vi "Add.vi"(7 "Service VI? (F)":bool, 8 "error in (no error)":errorcluster, 9 "RESTful VI configuration":T1={"Service VI Type"=enum."Web Method", "Load VI at statup"=TRUE, "Keep VI in memory"=TRUE, "Output type"=enum."Terminal", "Output format"=enum."XML", "Use headers"=TRUE, "Buffered"=TRUE, "eng_Load VI by name"=FALSE}, 10 "ProjectItem Refnum":refnum<vi>, 11 "NI_AB_API_RESTful in":refnum<class "NI_AB_API_RESTful.lvclass">) -> (0 "error out":errorcluster, 3 "NI_AB_API_RESTful out":refnum<class "NI_AB_API_RESTful.lvclass">)   [LabVIEW 2020, in "NI_AB_API_RESTful.lvclass"]
uses:
  <vilib>/AppBuilder/AB_API/RESTful/NI_AB_API_RESTful.lvclass
  <vilib>/AppBuilder/AB_API/RESTful/NI_AB_API_RESTful.lvclass/NI_AB_API_RESTful.ctl
  <vilib>/AppBuilder/AB_Classes/Build/AB_Build.lvclass
  <vilib>/AppBuilder/AB_Classes/Source/AB_Source.lvclass
  <vilib>/AppBuilder/AB_API/Build/NI_AB_API_Build.lvclass
  <vilib>/AppBuilder/AB_Classes/RESTful/AB_RESTfulWebService.lvclass
  e:/builds/penguin/labview/branches/2020/dev/dist/vi.lib/AppBuilder/AB_API/Targetfile/NI_AB_API_Targetfile.lvclass
  e:/builds/penguin/labview/branches/2020/dev/dist/vi.lib/AppBuilder/AB_API/Build/NI_AB_API_Build.lvclass
  e:/builds/penguin/labview/branches/2020/dev/dist/vi.lib/AppBuilder/AB_API/RESTful/NI_AB_API_RESTful.lvclass
  e:/builds/penguin/labview/branches/2020/dev/dist/vi.lib/AppBuilder/AB_Classes/WebService/AB_WebService.lvclass
  e:/builds/penguin/labview/branches/2020/dev/dist/vi.lib/AppBuilder/AB_Classes/TargetFile/AB_Targetfile.lvclass
  e:/builds/penguin/labview/branches/2020/dev/dist/vi.lib/AppBuilder/AB_Classes/Build/AB_Build.lvclass
  e:/builds/penguin/labview/branches/2020/dev/dist/vi.lib/AppBuilder/AB_Classes/RESTful/AB_RESTfulWebService.lvclass
  <vilib>/AppBuilder/AB_Classes/Source/VI/AB_Source_VI.lvclass
  e:/builds/penguin/labview/branches/2020/dev/dist/vi.lib/AppBuilder/AB_Classes/Source/AB_Source.lvclass
  e:/builds/penguin/labview/branches/2020/dev/dist/vi.lib/AppBuilder/AB_Classes/Source/VI/AB_Source_VI.lvclass
  <vilib>/AppBuilder/AB_Classes/Source/RESTfulVI/Configure_RESTfulVI/AB_RESTful_VIType.ctl
  <vilib>/AppBuilder/AB_Classes/Source/RESTfulVI/Configure_RESTfulVI/AB_RESTful_OutputType.ctl
  <vilib>/AppBuilder/AB_Classes/Source/RESTfulVI/Configure_RESTfulVI/AB_RESTful_OutputFormat.ctl
  <vilib>/AppBuilder/AB_Classes/Source/RESTfulVI/Configure_RESTfulVI/AB_RESTful_Configuration.ctl
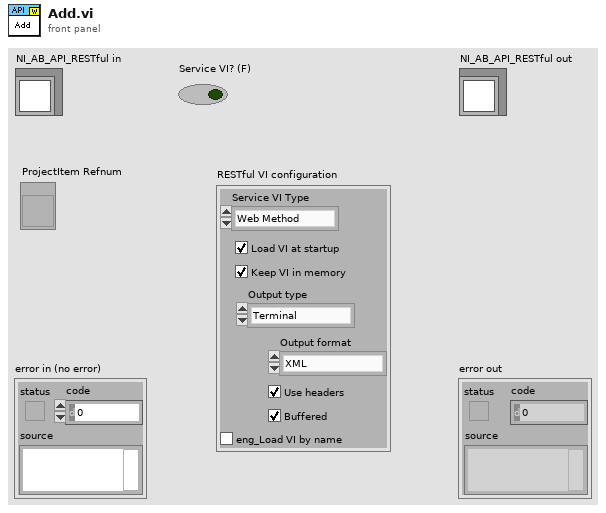
[diagram p1: front panel]
types:
  T1 = typedef "AB_RESTful_Configuration.ctl" = cluster{"Service VI Type":T2, "Load VI at statup":bool, "Keep VI in memory":bool, "Output type":T3, "Output format":T4, "Use headers":bool, "Buffered":bool, "eng_Load VI by name":bool}
  T2 = typedef "AB_RESTful_VIType.ctl" = enum32{"Web Method", "Auxiliary", "eng_Internal", "eng_Content"}
  T3 = typedef "AB_RESTful_OutputType.ctl" = enum32{"Terminal", "Stream"}
  T4 = typedef "AB_RESTful_OutputFormat.ctl" = enum32{"XML", "Text", "HTML", "JSON"}
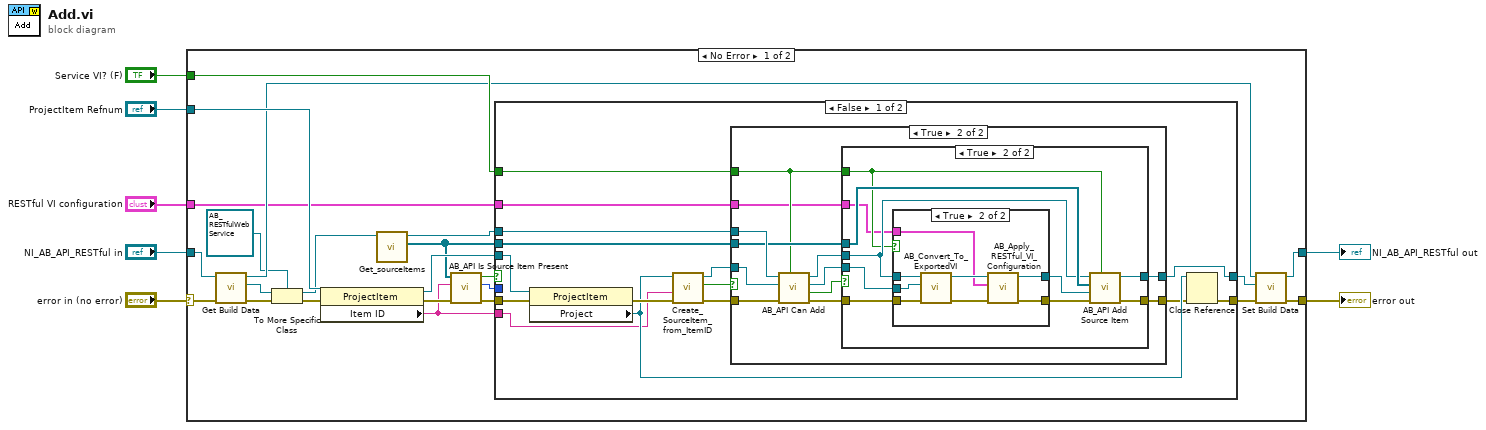
[diagram p0: block diagram]
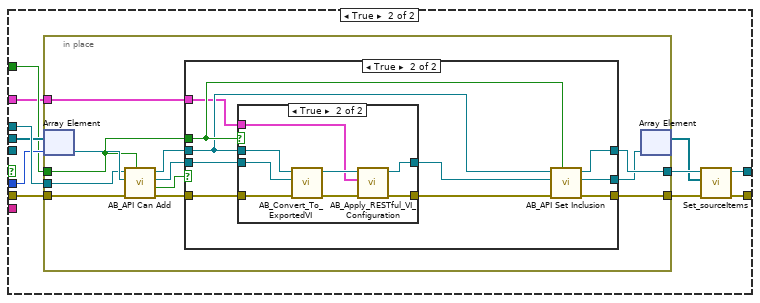
[diagram p5: hidden frame]
diagram:
  n1 = case shown="No Error" "error in (no error)" {
    selector: "error in (no error)" -> [w14 w129]
    tunnel: [w16 w129] -> w4
    tunnel: [w18 w128] -> w5
    tunnel: "NI_AB_API_RESTful in" -> [w19 w128]
    tunnel: "ProjectItem Refnum" -> [w30 _]
    tunnel: "Service VI? (F)" -> [w29 _]
    tunnel: "RESTful VI configuration" -> [w8 _]
    frame No Error {
      n2 = call <vilib>:"Get Build Data.vi"("error in (no error)"=w14, "NI_AB_API_Build in"=w19) -> ("error out"=w10:errorcluster, "AB_Build.lvclass"=w13:refnum<class "AB_Build.lvclass">, "NI_AB_API_Build out"=w20:refnum<class "NI_AB_API_RESTful.lvclass">)  [unwired: 7 in]
      n3 = To More Specific Class(target class=refnum<class "AB_RESTfulWebService.lvclass"> refnum ("AB_RESTfulWebService.lvclass"), reference=w13, error in=w10) -> (specific class reference=w12:refnum<class "AB_RESTfulWebService.lvclass">, error out=w9:errorcluster)
      n4 = property class="ProjectItem"(reference=w30, error in=w9) -> (reference out=w28:refnum<vi>, error out=w23:errorcluster, "Item ID"=w22:string)
      n5 = call <vilib>:"Get_sourceItems.vi"("Class in"=w12) -> ("sourceItems"=w27:refnum<class "AB_Source.lvclass">[], "Class out"=w26:refnum<class "AB_RESTfulWebService.lvclass">)  [unwired: 1 in, 8 out]
      n6 = call <vilib>:"AB_API Is Source Item Present.vi"("error in"=w23, "item ID"=w22, "source items"=w27) -> ("error out"=w24:errorcluster, "index"=w21:i32, "source item present?"=w25:bool)  [unwired: 3 in, 3 out]
      n7 = case shown="False" w25 {
        tunnel: w28 -> [w45 _]
        tunnel: [w41 w86] -> w17
        tunnel: [w37 w89] -> w15
        tunnel: w24 -> [w36 w88]
        tunnel: w26 -> [w35 w87]
        tunnel: w22 -> [w34 _]
        tunnel: w27 -> [w33 w85]
        tunnel: w21 -> [_ w84]
        tunnel: w29 -> [w32 w83]
        tunnel: w8 -> [w31 w82]
        frame False {
          n8 = property class="ProjectItem"(reference=w45, error in=w36) -> (error out=w44:errorcluster, "Project"=w39:refnum<vi>)  [unwired: 1 out]
          n9 = call <vilib>:"Create_SourceItem_from_ItemID.vi"("error in (no error)"=w44, "itemID"=w34, "Project Refnum"=w39) -> ("error out"=w42:errorcluster, "valid?"=w40:bool, "AB_Source out"=w43:refnum<class "AB_Source.lvclass">)  [unwired: 6 out]
          n10 = case shown="True" w40 {
            tunnel: w43 -> [_ w54]
            tunnel: w42 -> [w46 w52]
            tunnel: w35 -> [w47 w57]
            tunnel: [w47 w59] -> w41
            tunnel: [w46 w58] -> w38
            tunnel: w33 -> [_ w55]
            tunnel: w32 -> [_ w50]
            tunnel: w31 -> [_ w48]
            frame False {
            }
            frame True {
              n11 = call <vilib>:"AB_API Can Add.vi"("top tree? (true)"=w50, "error in (no error)"=w52, "AB_Source in"=w54, "Build in"=w57) -> ("error out"=w51:errorcluster, "can add?"=w49:bool, "AB_Source out"=w53:refnum<class "AB_Source.lvclass">, "Build out"=w56:refnum<class "AB_RESTfulWebService.lvclass">)  [unwired: 4 in]
              n12 = case shown="True" w49 {
                tunnel: w56 -> [w61 w64]
                tunnel: [w61 w69] -> w59
                tunnel: [w60 w70] -> w58
                tunnel: w51 -> [w60 w68]
                tunnel: w53 -> [_ w65]
                tunnel: w55 -> [_ w71]
                tunnel: w50 -> [_ w63]
                tunnel: w48 -> [_ w62]
                frame False {
                }
                frame True {
                  n13 = case shown="True" w63 {
                    tunnel: [w72 w77] -> w66
                    tunnel: [w73 w75] -> w67
                    tunnel: w64 -> [_ w79]
                    tunnel: w65 -> [w72 w81]
                    tunnel: w68 -> [w73 w80]
                    tunnel: w62 -> [_ w74]
                    frame False {
                    }
                    frame True {
                      n14 = call <vilib>:"AB_Convert_To_ExportedVI.vi"("error in (no error)"=w80, "Source in"=w81, "Build in"=w79) -> ("error out"=w76:errorcluster, "Exported VI out"=w78:refnum<class "AB_Source_VI.lvclass">)  [unwired: 7 out]
                      n15 = call <vilib>:"AB_Apply_RESTful_VI_Configuration.vi"("error in (no error)"=w76, "RESTful VI configuration"=w74, "VI in"=w78) -> ("error out"=w75:errorcluster, "VI out"=w77:refnum<class "AB_Source_VI.lvclass">)  [unwired: 7 in]
                    }
                  }
                  n16 = call <vilib>:"AB_API Add Source Item.vi"("top tree? (true)"=w63, "error in"=w67, "Source in"=w66, "source items"=w71, "Build in"=w64) -> ("error out"=w70:errorcluster, "Build out"=w69:refnum<class "AB_RESTfulWebService.lvclass">)  [unwired: 3 in, 2 out]
                }
              }
            }
          }
          n17 = Close Reference(reference=w39, error in (no error)=w38) -> (error out=w37:errorcluster)
        }
        frame True {
          n18 = in-place {
            in-place-border: [w104] -> w92
            in-place-border: w87 -> [w97]
            in-place-border: w88 -> [w101]
            in-place-border: [w103] -> w90
            in-place-border: w83 -> [w94]
            in-place-border: w82 -> [w93]
            n19 = in-place-array #1(w85, w84) -> (w99:refnum<class "AB_Source.lvclass">)
            n20 = call <vilib>:"AB_API Can Add.vi"("top tree? (true)"=w94, "error in (no error)"=w101, "AB_Source in"=w99, "Build in"=w97) -> ("error out"=w100:errorcluster, "can add?"=w95:bool, "AB_Source out"=w98:refnum<class "AB_Source.lvclass">, "Build out"=w96:refnum<class "AB_RESTfulWebService.lvclass">)  [unwired: 4 in]
            n21 = case shown="True" w95 {
              tunnel: [w105 w115] -> w103
              tunnel: [w107 w117] -> w104
              tunnel: w96 -> [w107 w109]
              tunnel: w98 -> [w106 w111]
              tunnel: w100 -> [w105 w113]
              tunnel: [w106 w116] -> w102
              tunnel: w94 -> [_ w114]
              tunnel: w93 -> [_ w108]
              frame False {
              }
              frame True {
                n22 = case shown="True" w114 {
                  tunnel: [w119 w121] -> w112
                  tunnel: w113 -> [w119 w125]
                  tunnel: [w118 w123] -> w110
                  tunnel: w111 -> [w118 w126]
                  tunnel: w109 -> [_ w127]
                  tunnel: w108 -> [_ w120]
                  frame False {
                  }
                  frame True {
                    n23 = call <vilib>:"AB_Convert_To_ExportedVI.vi"("error in (no error)"=w125, "Source in"=w126, "Build in"=w127) -> ("error out"=w122:errorcluster, "Exported VI out"=w124:refnum<class "AB_Source_VI.lvclass">)  [unwired: 7 out]
                    n24 = call <vilib>:"AB_Apply_RESTful_VI_Configuration.vi"("error in (no error)"=w122, "RESTful VI configuration"=w120, "VI in"=w124) -> ("error out"=w121:errorcluster, "VI out"=w123:refnum<class "AB_Source_VI.lvclass">)  [unwired: 7 in]
                  }
                }
                n25 = call <vilib>:"AB_API Set Inclusion.vi"("top tree? (true)"=w114, "error in (no error)"=w112, "Source in"=w110, "Build in"=w109) -> ("error out"=w115:errorcluster, "AB_Source_VI out"=w116:refnum<class "AB_Source.lvclass">, "AB_Build out"=w117:refnum<class "AB_RESTfulWebService.lvclass">)  [unwired: 5 in]
              }
            }
            n26 = in-place-array #1(w102) -> (w91:refnum<class "AB_Source.lvclass">[])  [unwired: 1 out]
          }
          n27 = call <vilib>:"Set_sourceItems.vi"("error in (no error)"=w90, "sourceItems"=w91, "Class in"=w92) -> ("error out"=w89:errorcluster, "Class out"=w86:refnum<class "AB_RESTfulWebService.lvclass">)  [unwired: 7 out]
        }
      }
      n28 = call <vilib>:"Set Build Data.vi"("error in (no error)"=w15, "AB_Build.lvclass"=w17, "NI_AB_API_Build in"=w20) -> ("error out"=w16:errorcluster, "NI_AB_API_Build out"=w18:refnum<class "NI_AB_API_RESTful.lvclass">)  [unwired: 7 in]
    }
    frame Error {
    }
  }
  "error out" <- w4
  "NI_AB_API_RESTful out" <- w5
